vi "Current System Status.vi"(7 "System Credentials":T1, 8 "error in":errorcluster, 11 "IP address":string) -> (0 "error out":errorcluster, 1 "Requires Update?":string, 2 "ImageTitle":string, 3 "Firmware Version":string)   [LabVIEW 2020]
uses:
  Controls/System Credentials.ctl
  <vilib>/nisyscfg/Get Installed Set.vi
  <vilib>/nisyscfg/Close (System).vi
  <resource>/objmgr/nisysapi.rc
  <vilib>/nisyscfg/nisyscfg.lvlib
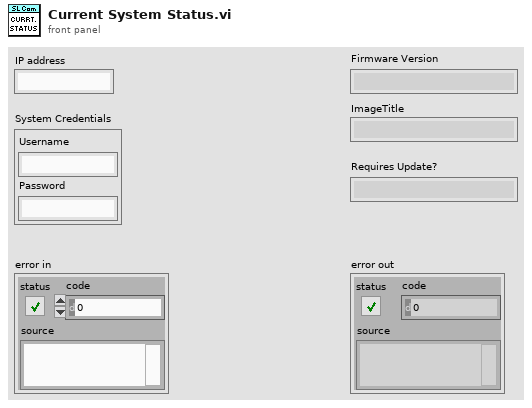
[diagram p1: front panel]
types:
  T1 = typedef "System Credentials.ctl" = cluster{"Username":string, "Password":string}
  T2 = typedef "nisyscfg.lvlib/Software Set 1.2.ctl" = cluster{"information":T3, "items":T3[], "add-ons":T3[]}
  T3 = typedef "nisyscfg.lvlib/Software 1.2.ctl" = cluster{"title":string, "description":string, "ID":string, "version":string, "component type":T4}
  T4 = typedef "nisyscfg.lvlib/Component Type.ctl" = u32
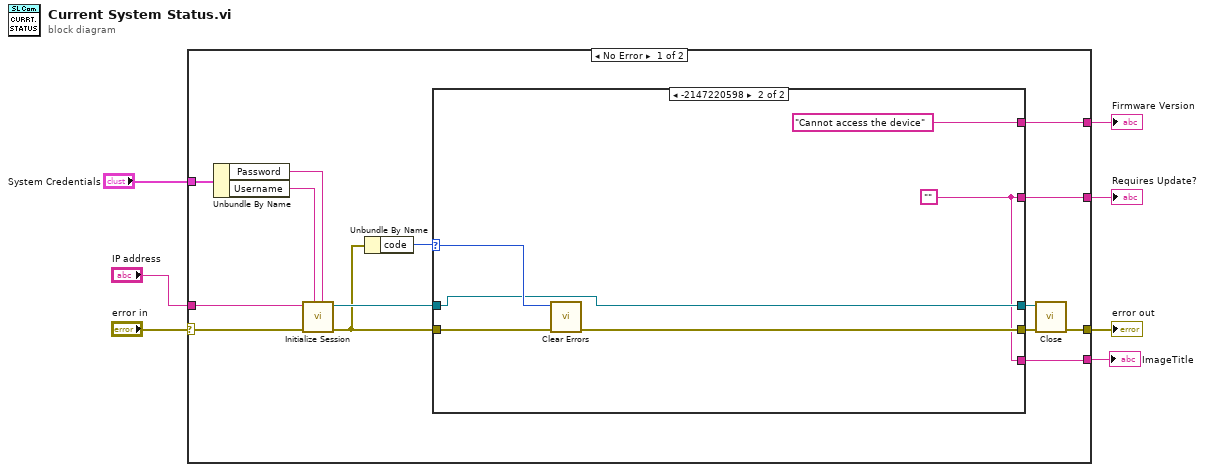
[diagram p0: block diagram]
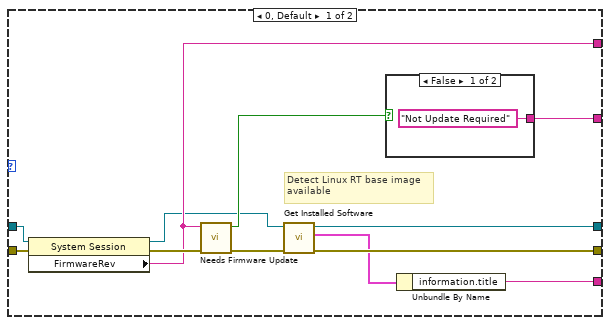
[diagram p2: hidden frame]
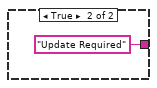
[diagram p3: hidden frame]
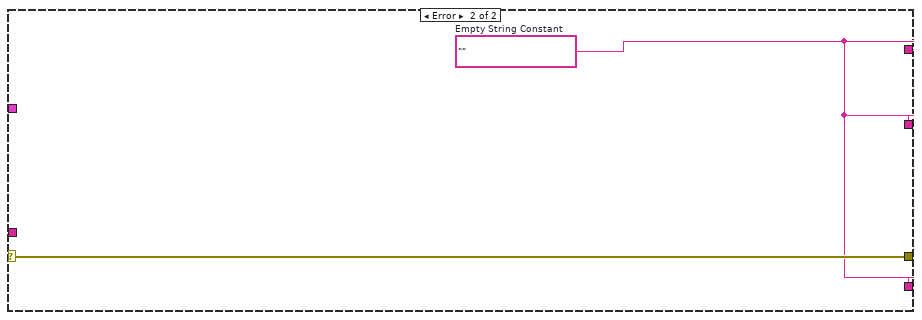
[diagram p4: hidden frame]
diagram:
  n1 = case shown="No Error" "error in" {
    selector: "error in" -> [w16 w43]
    tunnel: [w21 w43] -> w7
    tunnel: "IP address" -> [w20 _]
    tunnel: [w18 w42] -> w5
    tunnel: [w17 w42] -> w4
    tunnel: [w13 w42] -> w2
    tunnel: "System Credentials" -> [w10 _]
    frame No Error {
      n2 = Unbundle By Name(w10) -> ("Password"=w8:string, "Username"=w9:string)
      n3 = call <vilib>:"Initialize Session.vi"("Password"=w8, "User Name"=w9, "error in (no error)"=w16, "Target (localhost)"=w20) -> ("error out"=w12:errorcluster, "Session out"=w19:refnum<k21>)  [unwired: 6 in]
      n4 = Unbundle By Name(w12) -> ("code"=w11:i32)
      n5 = case shown="-2147220598" w11 {
        selector: w11 -> [_ w40]
        tunnel: w12 -> [w33 w41]
        tunnel: w19 -> [w32 w39]
        tunnel: [w29 w36] -> w18
        tunnel: [w28 "Cannot access the device" ("title")] -> w17
        tunnel: [w26 w39] -> w15
        tunnel: [w25 w38] -> w14
        tunnel: [w22 w36] -> w13
        frame 0, Default {
          # "Detect Linux RT base image\navailable"
          n6 = property class="System Session"(reference=w32, error in=w33) -> (reference out=w27:refnum<k21>, error out=w31:errorcluster, "FirmwareRev"=w28:string)
          n7 = call "Needs Firmware Update.vi"("error in (no error)"=w31, "FirmwareRev"=w28) -> ("error out"=w24:errorcluster, "Update?"=w30:bool)  [unwired: 8 in]
          n8 = call-poly <vilib>:"Get Installed Software.vi"("error in (no error)"=w24, "Session in"=w27) -> ("error out"=w25:errorcluster, "Software Set"=w23:T2, "Session out"=w26:refnum<k21>)  [unwired: 7 in]
          n9 = case shown="False" w30 {
            tunnel: ["Not Update Required" ("Requires Update?") "Update Required" ("Requires Update?")] -> w29
            frame False {
            }
            frame True {
            }
          }
          n10 = Unbundle By Name(w23) -> ("information.title"=w22:string)
        }
        frame -2147220598 {
          w36 = "" ("Requires Update?")
          n11 = call <vilib>:"Clear Errors.vi"("error in (no error)"=w41, "specific error code to clear (0: all)"=w40) -> ("error out"=w38:errorcluster)  [unwired: 4 in, 1 out]
        }
      }
      n12 = call-poly <vilib>:"Close.vi"("error in (no error)"=w14, "Session in"=w15) -> ("error out"=w21:errorcluster)  [unwired: 9 in]
    }
    frame Error {
      w42 = ""  # Empty String Constant
    }
  }
  "error out" <- w7
  "Firmware Version" <- w4
  "Requires Update?" <- w5
  "ImageTitle" <- w2
